vi "ParseReply.vi"(8 "Parent":string, 11 "Console":string) -> (1 "PythonFiles":string[](array[string]), 2 "Folders":string[](array[string]), 3 "all files":string[](array[string]))   [LabVIEW 2022 SP3]
uses:
  <vilib>/Utility/error.llb/Trim Whitespace One-Sided.vi
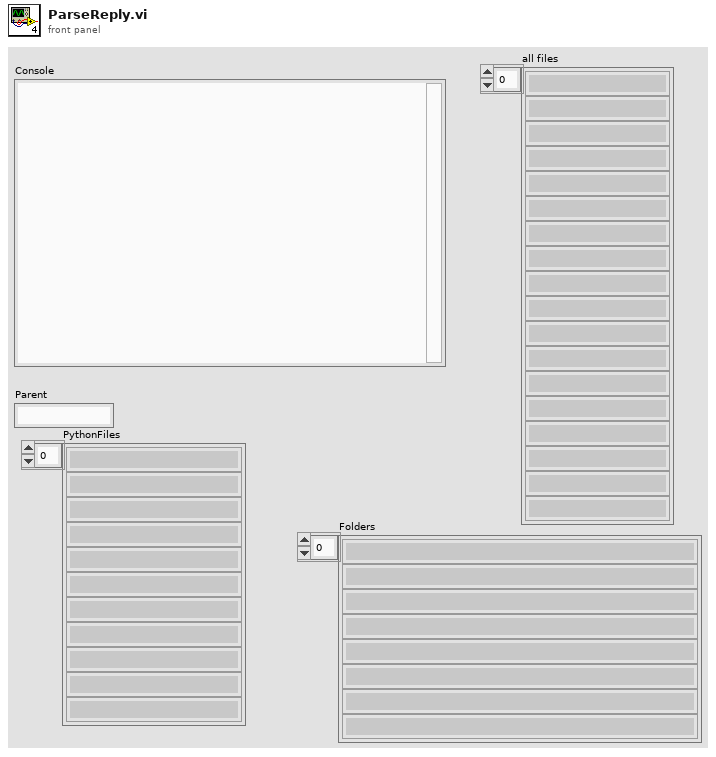
[diagram p1: front panel]
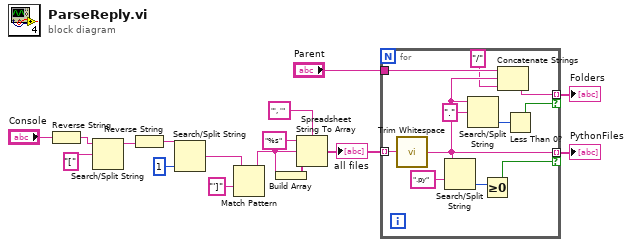
[diagram p0: block diagram]
diagram:
  n1 = Reverse String(1:"Console") -> (0:w6:string)
  n2 = Search/Split String(string=w6, search string/char (-)="[" ("regular expression")) -> (substring before match=w5:string)  [unwired: 1 in, 2 out]
  n3 = Reverse String(1:w5) -> (0:w3:string)
  n4 = Search/Split String(string=w3, offset (0)=1) -> (match + rest of string=w2:string)  [unwired: 1 in, 2 out]
  n5 = Match Pattern(string=w2, regular expression="']") -> (before substring=w9:string)  [unwired: 1 in, 3 out]
  n6 = Build Array(w9) -> (w10:string[])
  n7 = Spreadsheet String To Array(delimiter (Tab)="', '", format string="%s", spreadsheet string=w9, array type (2D Dbl)=w10) -> (array=w13:string[])
  "all files" <- w13
  n8 = for {
    tunnel: w13 -> [w27] mode=indexing
    tunnel: [w18] -> w14 mode=indexing if=w24
    tunnel: [w19] -> w15 mode=indexing if=w21
    tunnel: "Parent" -> [w20]
    n9 = call <vilib>:"Trim Whitespace.vi"("string"=w27) -> ("trimmed string"=w18:string)  [unwired: 1 in]
    n10 = Search/Split String(string=w18, search string/char (-)=".py" ("regular expression")) -> (offset of match=w25:i32)  [unwired: 1 in, 2 out]
    n11 = Search/Split String(string=w18, search string/char (-)=".") -> (offset of match=w22:i32)  [unwired: 1 in, 2 out]
    n12 = Greater Or Equal To 0?(x=w25) -> (x >= 0?=w24:bool)
    n13 = Concatenate Strings(w20, w18, "/" ("search string/char (-)")) -> (w19:string)
    n14 = Less Than 0?(x=w22) -> (x < 0?=w21:bool)
  }
  "Folders" <- w15
  "PythonFiles" <- w14
